vi "GetExptDevices.vi"() -> ()   [LabVIEW 2020]
uses:
  Shared/MySQL/Preset Query Enum.ctl
panel:
  in  "stop":bool
  out "Multicolumn Listbox":i32[](listbox)
  in  "Expt name / MCIP/ Variable/Preset Name":string
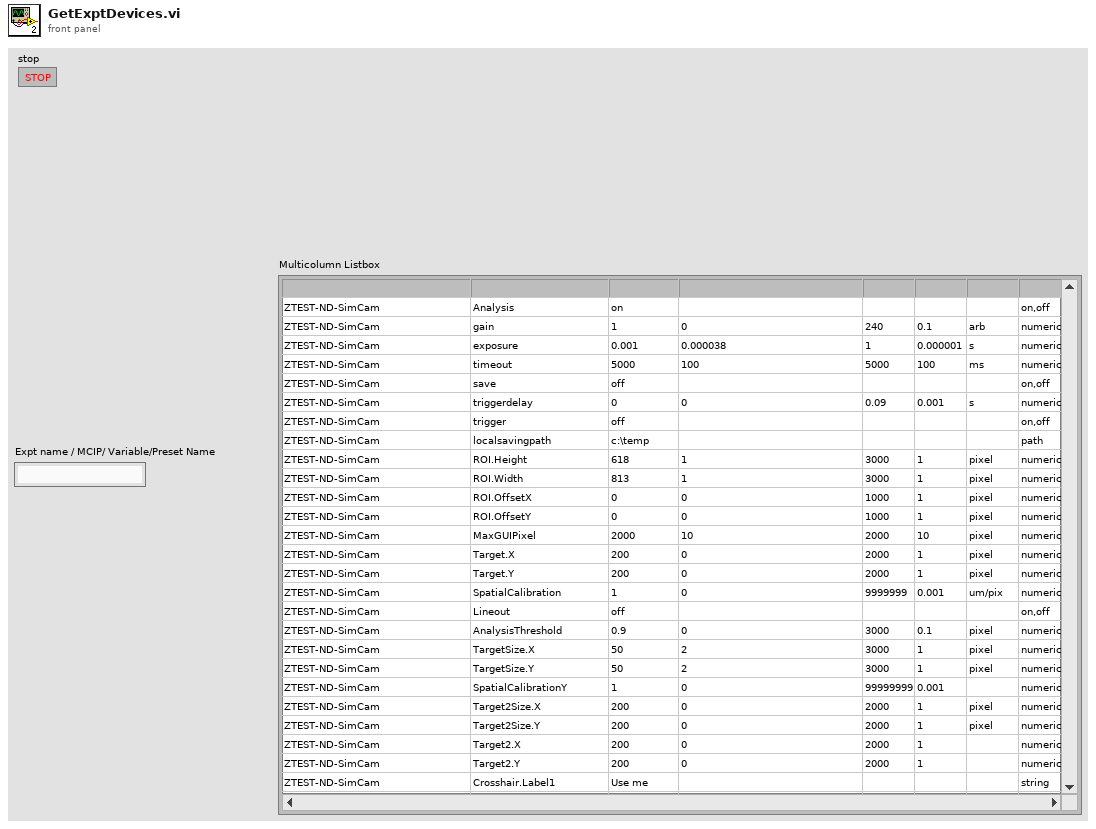
[diagram p1: front panel]
types:
  T1 = typedef "Preset Query Enum.ctl" = enum16{"Get Locations", "Get all IPs and MACs", "Get classes", "Get expt variables to set at scanstart for particular device", "Get expt devices and variables with start values", "Get expt devices and variables (with data to get)", "Get expt devices with data to get", "Get Expt devices and GUIs", "Get all devices basic properties", "Get Virtual Devices Core Info", "Get Expt names", "Get experiment basic properties", "Get experiment alarm variables", "Get MC Ports", "Get device network comm port", "Get devicetype lvclass path", "Get basic device properties", "Get Init Order", "Get all setable variables of a device", "Get device variable aliases", "Get force values of all settable variables", "Get all variables of a devicetype", "Get all variables of a device", "Get plotter details", "Get Saved Scans", "Get Scan Info", "GetGeneralGUIs", "Get expt for plotter", "Get plotter IDs from expt", "Get all devices", "Get all Virtual Devices", "Get all aliases", "Get variable and device info for Virtual Device", "GetItemLocatorIP", "Get IPs for GUIs", "Get DeviceType from Device", "GetLocalPortRange", "GetDevicePresetVariables", "Get Device Configuration", "GetAllPresetNames", "GetAllConfigurationNames", "GetPresetDeviceNames", "GetDeviceAliases", "GetDevicesOfClass"}
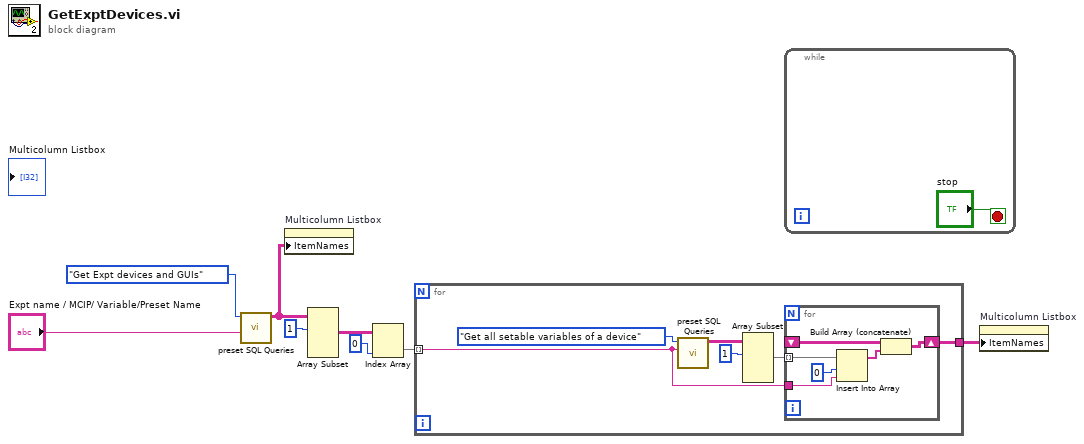
[diagram p0: block diagram]
diagram:
  n1 = call "preset SQL Queries.vi"("Expt name / MCIP/ Variable/Preset Name"="Expt name / MCIP/ Variable/Preset Name", "Preset Query"=Preset_Query_Enum."Get Expt devices and GUIs") -> ("data"=w6:string[][])  [unwired: 7 in, 2 out]
  n2 = property on="Multicolumn Listbox" class="MCListbox (strict)"("ItemNames"=w6) -> ()  [unwired: 2 in, 2 out]
  n3 = Array Subset(array=w6, index (row)=1 ("disabled index (col)")) -> (w4:string[][])  [unwired: 3 in]
  n4 = Index Array(array=w4, index (col)=0 ("disabled index (col)")) -> (element=w2:string[])  [unwired: 1 in]
  n5 = for {
    tunnel: w2 -> [w13] mode=indexing
    tunnel: [w12] -> w1
    n6 = call "preset SQL Queries.vi"("Device/Devicetype name\n/Plotter.id/ScanName#"=w13, "Preset Query"=Preset_Query_Enum."Get all setable variables of a device") -> ("data"=w11:string[][])  [unwired: 7 in, 2 out]
    n7 = Array Subset(array=w11, index (row)=1) -> (w9:string[][])  [unwired: 3 in]
    n8 = for {
      tunnel: w13 -> [w20]
      shift-right: [w17] -> w12
      shift-left: _ -> [w16]
      tunnel: w9 -> [w15] mode=indexing
      n9 = Insert Into Array(array=w15, index=0, new element=w20) -> (w18:string[])
      n10 = Build Array (concatenate)(w16, w18) -> (w17:string[][])
    }
  }
  n11 = while {
    stop <- "stop" stop-if-true
  }
  n12 = property on="Multicolumn Listbox" class="MCListbox (strict)"("ItemNames"=w1) -> ()  [unwired: 2 in, 2 out]
